vi "sv_Build Octave Info (N Ch).vi"(0 "scaled signals":waveform(dbl)[](array[waveform]), 5 "1/n octave settings":T2={"standard"=enum."ANSI S1.11", "bandwidth"=enum."1/3 octave"}, 7 "band number":cluster{"low band":i32, "high band":i32}, 11 "error in (no error)":errorcluster) -> (3 "octave info":T3[](array[typedef]) {"engineering units" items=["custom..."=0, "V"=1, "A"=21, "C"=30, "pC"=31, "s"=32, "-"=29, "Pa"=2, "N"=20, "g"=3, "m/s^2"=4, "m/s"=5, "m"=6, "mm/s"=12, "mm"=13, "micron/s"=14, "micron"=15, "in/s^2"=7, "in/s"=8, "in"=9, "mil/s"=10, "mil"=11, "rad/s^2"=16, "rad/s"=17, "rad"=18, "deg/s^2"=26, "deg/s"=27, "deg"=28, "RPM"=22, "cycle/s^2"=23, "Hz"=24, "cycle"=25, "strain"=19]; "dB reference" format="%.2e"; "weighting filter" items=["Linear", "A-weighting", "B-weighting", "C-weighting", "ITU-R 468-4", "Dolby", "CCITT", "C-message", "Wb", "Wc", "Wd", "We", "Wf", "Wh", "Wj", "Wk", "Wm", "AES17 20 kHz lowpass", "AES17 40 kHz lowpass", "AES17 20 kHz highpass", "AES17 40 kHz highpass"]}, 4 "scaled signals":waveform(dbl)[](array[waveform]), 6 "dup 1/n octave settings":T2={"standard"=enum."ANSI S1.11", "bandwidth"=enum."1/3 octave"}, 8 "dup band number":cluster{"low band":i32, "high band":i32}, 15 "error out":errorcluster)   [LabVIEW 2017, in "SoundVib_Octave_2014 standard.lvlib"]
uses:
  <vilib>/addons/Sound and Vibration/svt_Octave/SoundVib_Octave_2014 standard.lvlib
  <vilib>/addons/_NISVFA/_Shared subVIs/Controls/svc_Octave Standard.ctl
  <vilib>/addons/_NISVFA/_Shared subVIs/Controls/svc_Octave Info.ctl
  <vilib>/addons/_NISVFA/_Shared subVIs/Controls/svc_Weighting Filter Text Ring.ctl
  <vilib>/addons/_NISVFA/_Shared subVIs/Controls/svc_Engineering Units Text Ring.ctl
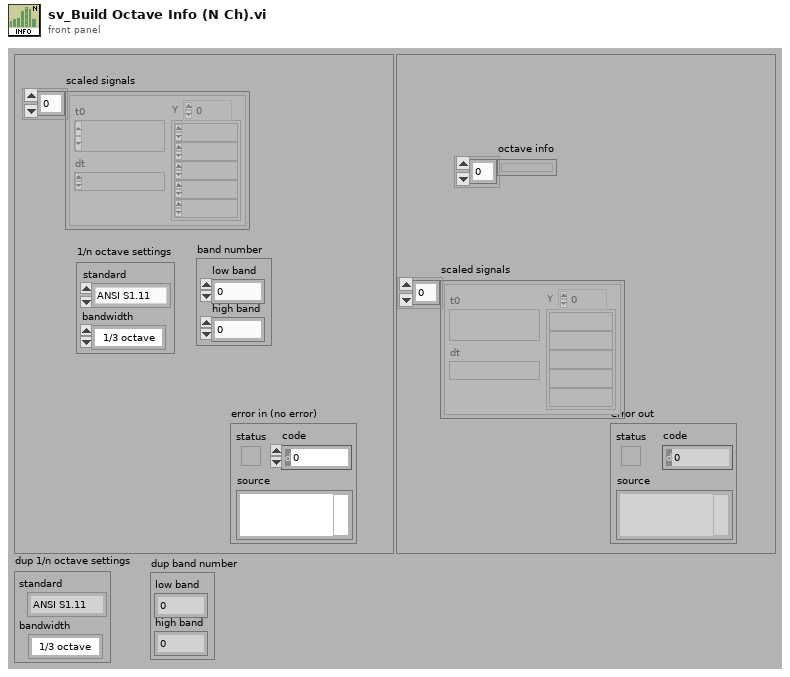
[diagram p1: front panel]
types:
  T1 = typedef "svc_Octave Standard.ctl" = enum16{"ANSI S1.11", "IEC 61260"}
  T2 = cluster{"standard":T1, "bandwidth":enum16{"1 octave", "1/3 octave", "1/6 octave", "1/12 octave", "1/24 octave"}}
  T3 = typedef "svc_Octave Info.ctl" = cluster{"standard":T1, "bandwidth":enum16{"1 octave", "1/3 octave", "1/6 octave", "1/12 octave", "1/24 octave"}, "low band":i32, "high band":i32, "weighting filter":T4, "dB reference":dbl, "dB On":bool, "unit label":string, "channel name":string, "description":string, "engineering units":T5, "custom label":string, "spectrum type":enum16{"power", "magnitude"}, "spectral density":bool, "filters settled":bool}
  T4 = typedef "svc_Weighting Filter Text Ring.ctl" = u16
  T5 = typedef "svc_Engineering Units Text Ring.ctl" = u16
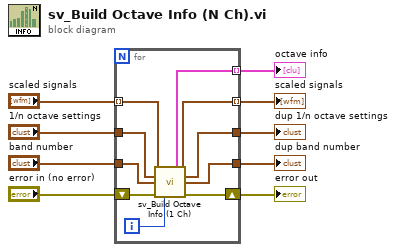
[diagram p0: block diagram]
diagram:
  n1 = for {
    tunnel: "scaled signals" -> [w18] mode=indexing
    tunnel: [w19] -> w8 mode=indexing
    shift-right: [w16] -> w4
    shift-left: "error in (no error)" -> [w17]
    tunnel: "1/n octave settings" -> [w15]
    tunnel: "band number" -> [w14]
    tunnel: [w13] -> w3
    tunnel: [w12] -> w2
    tunnel: [w11] -> w1 mode=indexing
    i -> [w10]
    n2 = call <vilib>:"sv_Build Octave Info (1 Ch).vi"("scaled signal [EU]"=w18, "1/n octave settings"=w15, "band number"=w14, "error in (no error)"=w17, "channel index"=w10) -> ("octave info"=w11:T3, "dup scaled signal [EU]"=w19:waveform(dbl), "dup 1/n octave settings"=w13:T2, "dup band number"=w12:cluster{"low band":i32, "high band":i32}, "error out"=w16:errorcluster)  [unwired: 6 in]
  }
  "octave info" <- w1
  "error out" <- w4
  "scaled signals" <- w8
  "dup 1/n octave settings" <- w3
  "dup band number" <- w2
